vi "fit_3_gauss.vi"(8 "initial parameters":dbl[](array[numeric])=[0.1, 2.0, 0.5, 0.1, 6.0, 0.5, 5.0], 10 "y Array":dbl[](array[numeric]), 11 "x Array":dbl[](array[numeric])) -> (0 "best fit parameters":dbl[](array[numeric]), 1 "XY Graph":cluster{dbl[], dbl[]}[](graph), 2 "Peak 3 Amp":dbl, 3 "Peak 1 Amp":dbl)   [LabVIEW 2011]
uses:
  <vilib>/gmath/NumericalOptimization/Nonlinear Curve Fit LM.vi
  <vilib>/gmath/NI_Gmath.lvlib
panel:
  out "error out":errorcluster
  in  "termination":cluster{"max iteration":i32, "tolerance":dbl}={"max iteration"=1000, "tolerance"=1e-09}
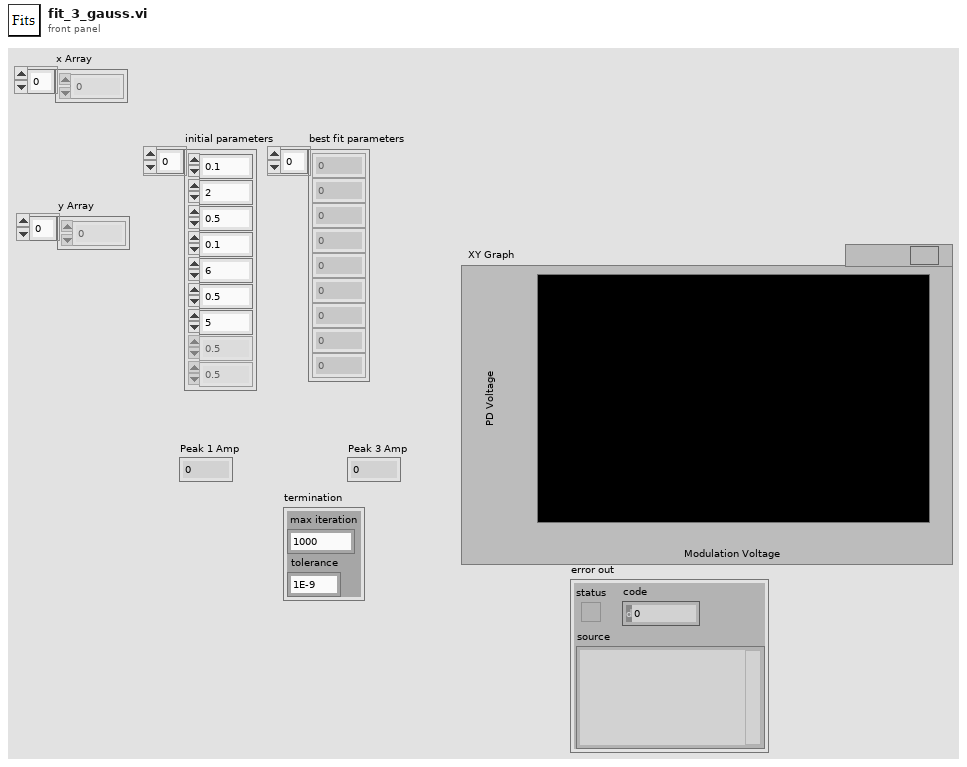
[diagram p1: front panel]
types:
  T1 = cluster{"x Array":dbl[], "best nonlinear fit":dbl[]}
  T2 = cluster{"x Array":dbl[], "best nonlinear fit":dbl[]}[]
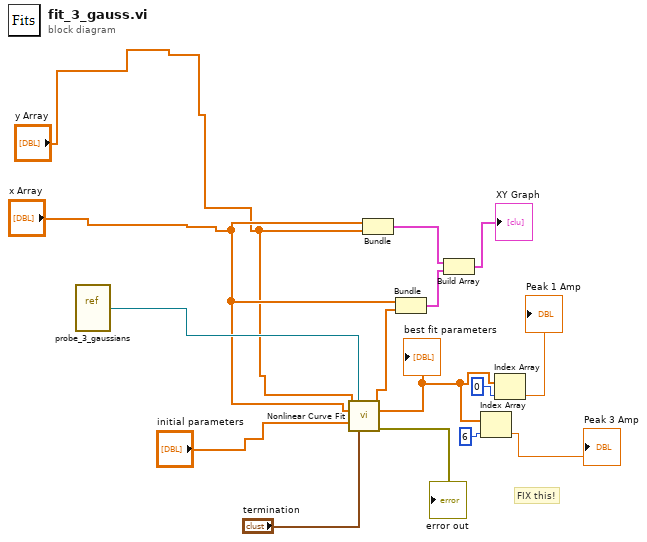
[diagram p0: block diagram]
diagram:
  # "FIX this!"
  n1 = vi-ref "probe_3_gaussians.vi"() -> (w10:refnum<vi>)
  n2 = call-poly <vilib>:"Nonlinear Curve Fit.vi"("Y"="y Array", "f(x,a)"=w10, "X"="x Array", "initial parameters"="initial parameters", "termination"="termination") -> ("best nonlinear fit"=w13:dbl[], "best fit parameters"=w5:dbl[], "error out"=→"error out":errorcluster)  [unwired: 5 in, 3 out]
  "best fit parameters" <- w5
  n3 = Bundle("x Array"="x Array", "y Array"="y Array") -> (w15:cluster{"x Array":dbl[], "y Array":dbl[]})  [unwired: 1 in]
  n4 = Bundle("x Array"="x Array", "best nonlinear fit"=w13) -> (w8:T1)  [unwired: 1 in]
  n5 = Build Array(w15, w8) -> (→"XY Graph":T2)
  n6 = Index Array(array=w5, index=6) -> (element=→"Peak 3 Amp":dbl)
  n7 = Index Array(array=w5, index=0) -> (element=→"Peak 1 Amp":dbl)
